vi "Calculate Directory Size (recursive).vi"(1 "Directory":string, 2 "Directory Tree":T1) -> (0 "Directory Size":u64)   [LabVIEW 2020, in "AoC 2022.lvlib"]
uses:
  AoC 2022.lvlib
  Directory Tree.ctl
  Directory Contents.ctl
  File.ctl
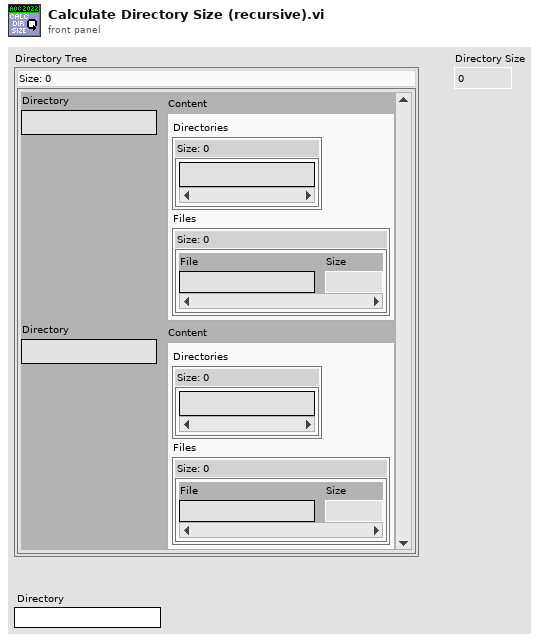
[diagram p1: front panel]
types:
  T1 = typedef "AoC 2022.lvlib/Directory Tree.ctl" = map{string, T2}
  T2 = typedef "AoC 2022.lvlib/Directory Contents.ctl" = cluster{"Directories":set{string}, "Files":T3}
  T3 = typedef "AoC 2022.lvlib/File.ctl" = map{string, u64}
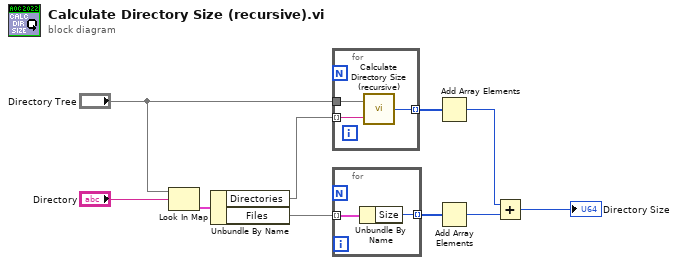
[diagram p0: block diagram]
diagram:
  n1 = Look In Map(map="Directory Tree", key="Directory") -> (value=w9:T2)  [unwired: 1 in, 1 out]
  n2 = Unbundle By Name(w9) -> ("Directories"=w2:set{string}, "Files"=w8:T3)
  n3 = for {
    tunnel: w2 -> [w13] mode=indexing
    tunnel: "Directory Tree" -> [w12]
    tunnel: [w11] -> w1 mode=indexing
    n4 = call "Calculate Directory Size (recursive).vi"("Directory"=w13, "Directory Tree"=w12) -> ("Directory Size"=w11:u64)
  }
  n5 = for {
    tunnel: w8 -> [w15] mode=indexing
    tunnel: [w14] -> w7 mode=indexing
    n6 = Unbundle By Name(w15) -> ("Size"=w14:u64)
  }
  n7 = Add Array Elements(numeric array=w1) -> (sum=w4:u64)
  n8 = Add Array Elements(numeric array=w7) -> (sum=w5:u64)
  n9 = Add(x=w4, y=w5) -> (x+y=→"Directory Size":u64)
